vi "HapticSTM_raw.vi"() -> ()   [LabVIEW 2019]
uses:
  <userlib>/HapticSTM/HapticSTM.lvlib
  SubVIs/GlobalClicksHeight_raw.vi
  <userlib>/Nanonis Prog Interface V5/Nanonis Prog Interface.lvlib
panel:
  in  "Version?":bool
  in  "Setpoint (pA)":dbl=100.0
  in  "Depth (pA)":dbl=280.0
  in  "Shift (in)":dbl format="%.1f"
  in  "Hardness":dbl=0.7 format="%.1f"
  in  "Z Write?":bool
  out "function return":i32
  in  "Scaling?":bool
  out "Setpoint (pA)":dbl
  in  "Maximum (pA)":dbl=7000.0
  out "Filtered Current (pA)":dbl format="%.1f"
  out "Current (pA)":dbl format="%.1f"
  out "Oy":dbl
  out "Ox":dbl
  out "W":dbl
  out "H":dbl
  out "Z Write":dbl format="%^.1e"
  in  "Planing?":bool
  out "Button":bool
  out "Fy":dbl format="%.1f"
  out "Fz":dbl format="%.1f"
  out "Fx":dbl format="%.1f"
  out "x":dbl format="%.1f"
  out "y":dbl format="%.1f"
  out "z":dbl format="%0.1f"
  in  "Mode":u16(ring) items=["Log w/ Exp Z", "Log w/ Lin Z"]
  in  "Reset Clicks":bool
  out "Clicks":i32
  in  "STOP":bool
  in  "START":bool
  out "Seq":i32
  out "SeqString":string
  out "Raw and Scaled Z Positions":cluster{"X":dbl, "Y":dbl, "Z pen":dbl, "Z":dbl}(graph)
  out "Scaled Force and Current":T1(graph)
  # "Super Ultra Mega Haptic STM Controller 3000"
  # "Haptic Pen"
  # "Nanonis"
  # "Position"
  # "Z Controller"
  # "Force"
  # "Frame"
  # "Surface"
  # "Options"
  # "Addons"
  # "Test Data"
  # "Live"
  # "Small"
  # "Large"
  # "Current"
  # "No"
  # "Yes"
  # "Planing"
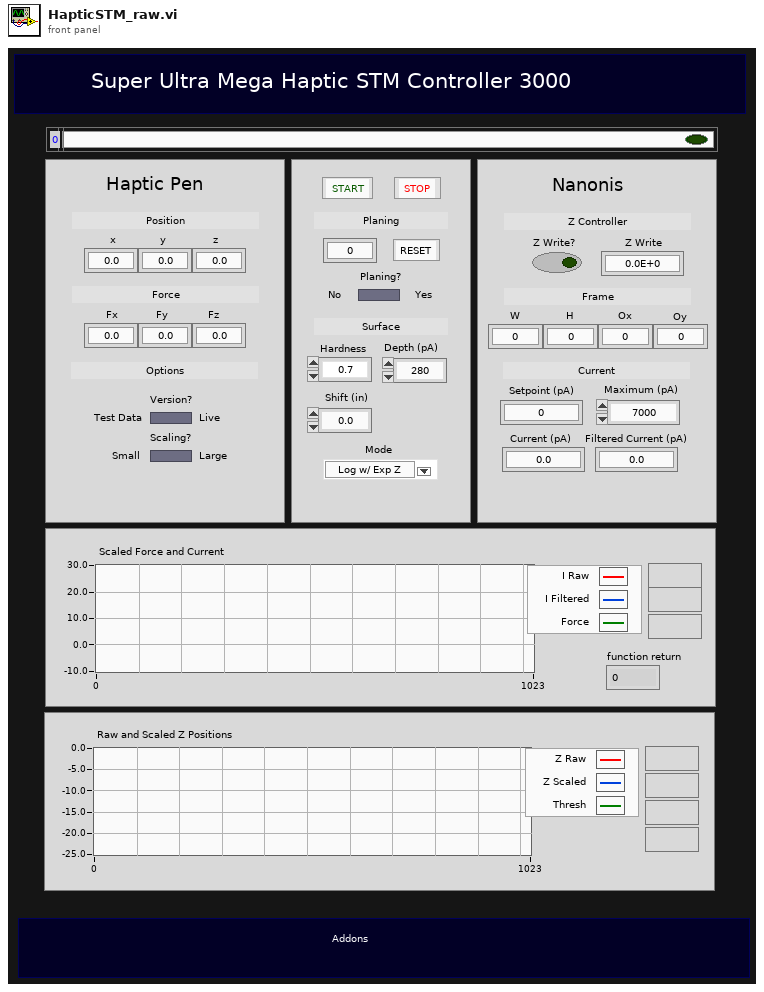
[diagram p1: front panel]
types:
  T1 = cluster{"Current (pA)":dbl, "Filtered Current (pA)":dbl, dbl}
  T2 = cluster{"Size (m)":cluster{"Width":sgl, "Height":sgl}, "Center coordinates (m)":cluster{"Xc":sgl, "Yc":sgl}}
  T3 = cluster{"Position":cluster{"X":dbl, "Y":dbl, "Zpen":dbl}, void, "y scaled (m)":dbl}
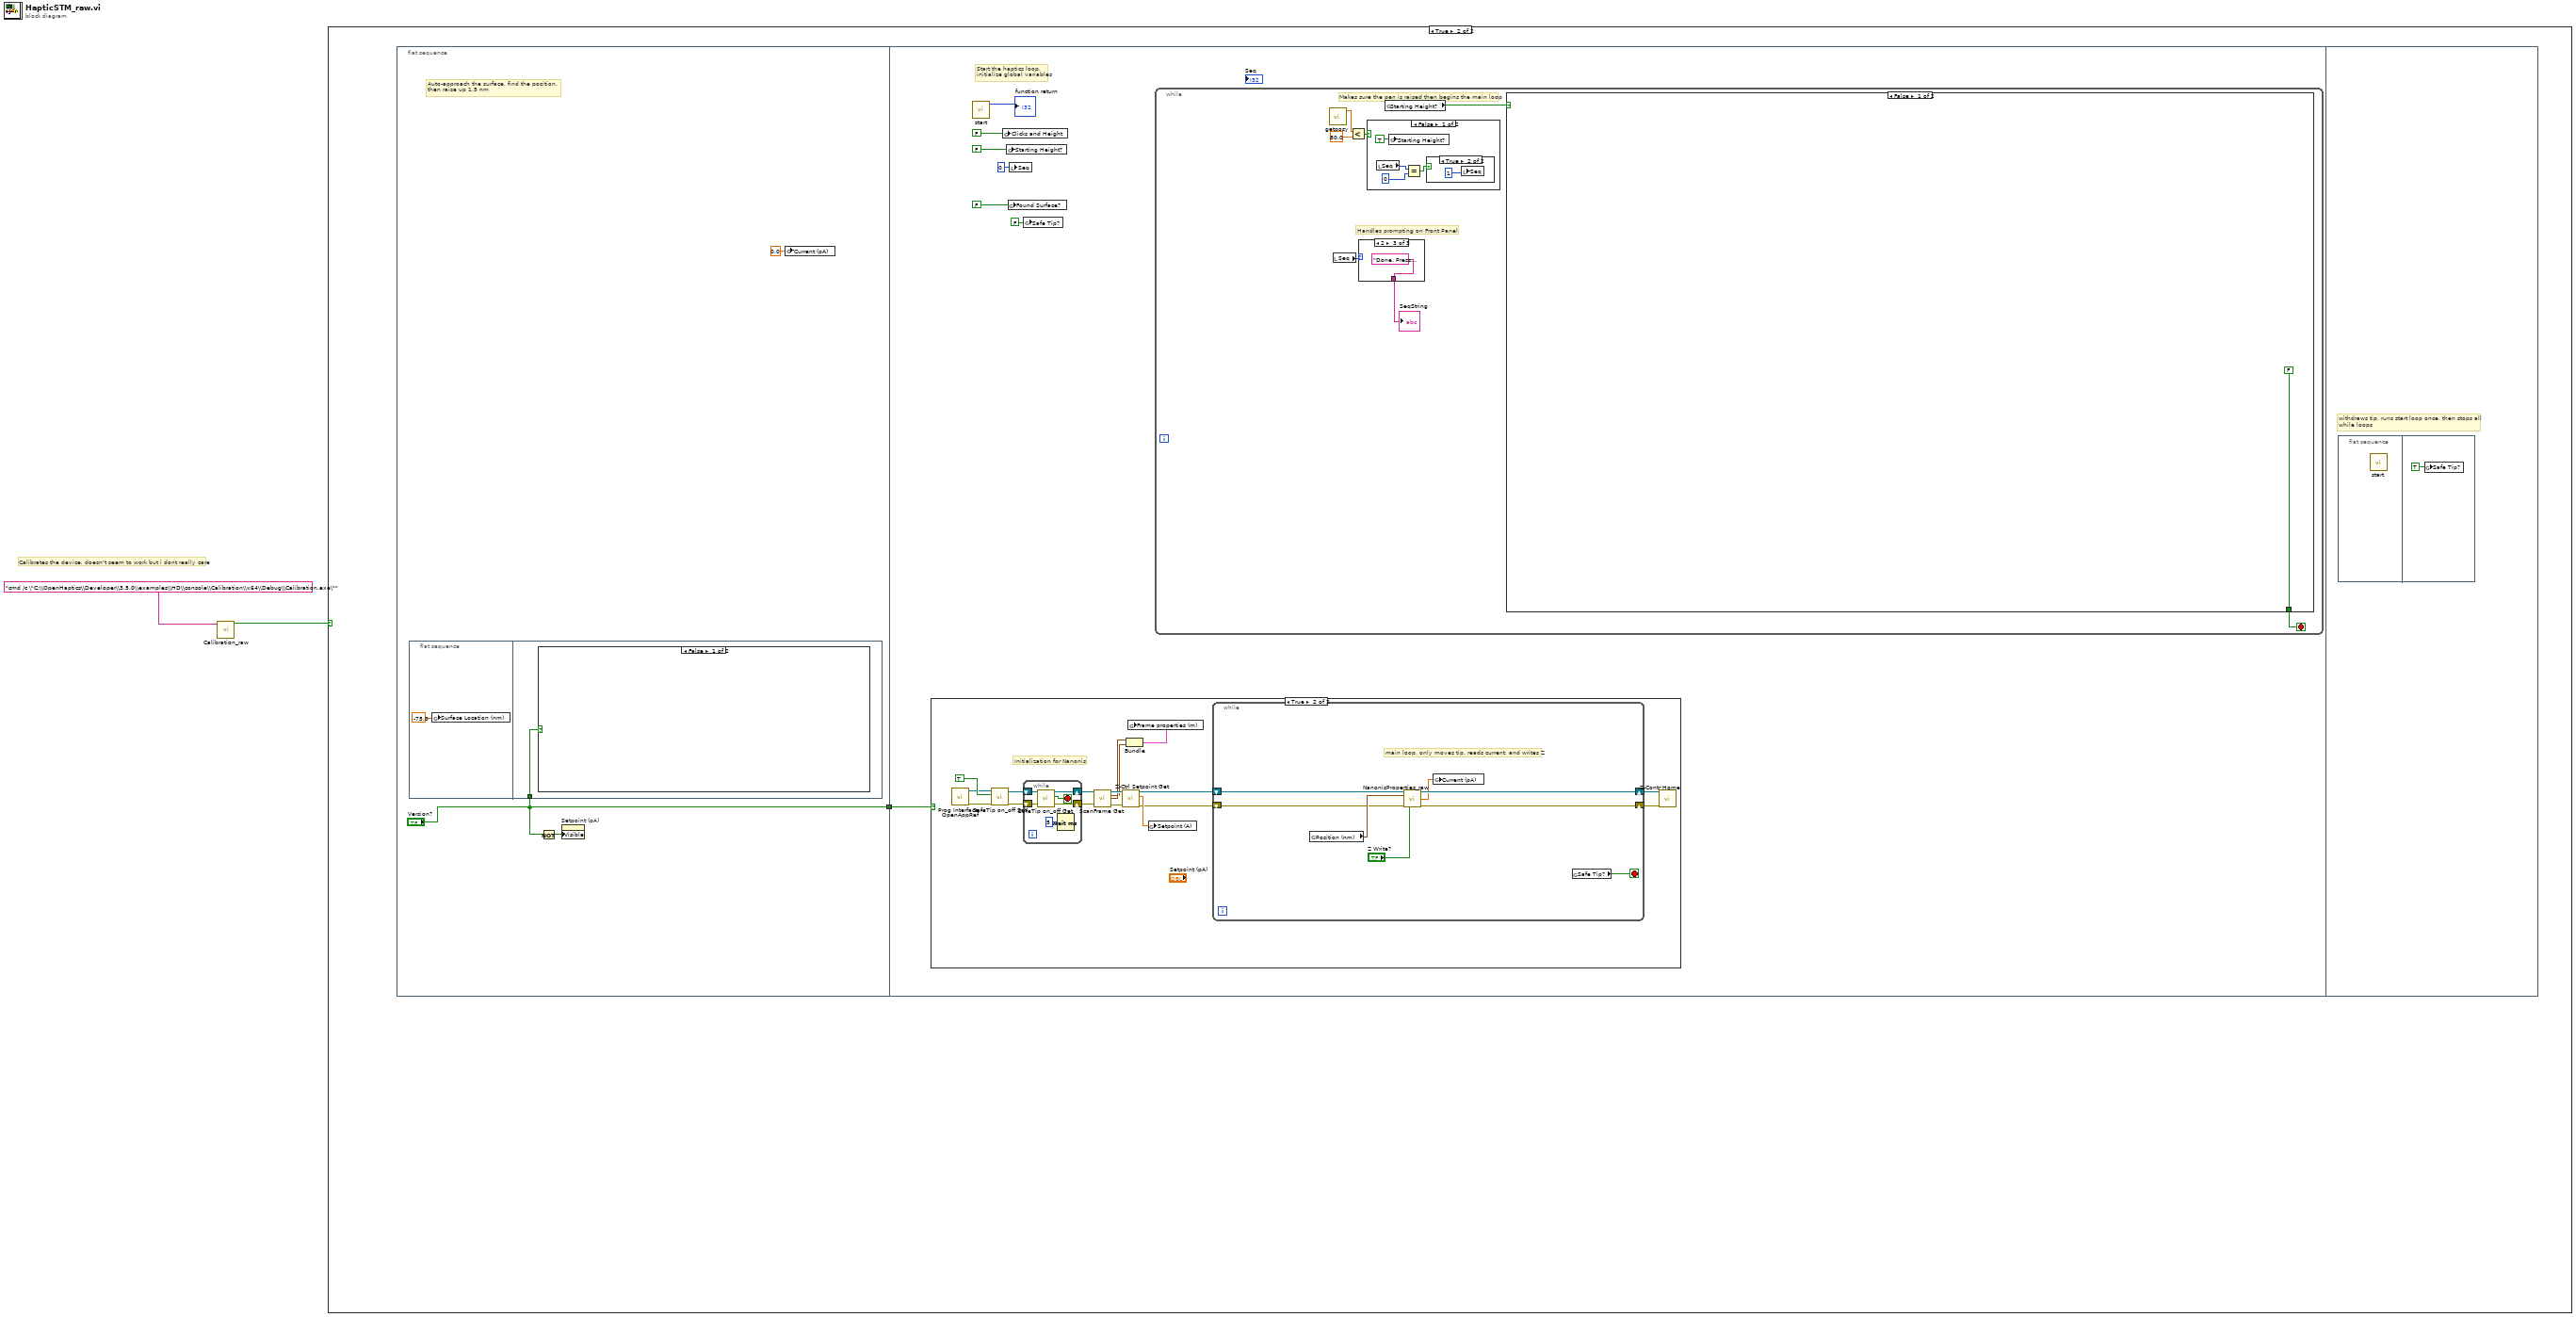
[diagram p0: block diagram]
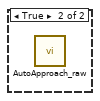
[diagram p3: hidden frame]
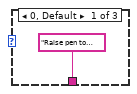
[diagram p5: hidden frame]
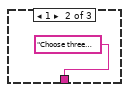
[diagram p6: hidden frame]
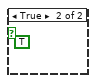
[diagram p8: hidden frame]
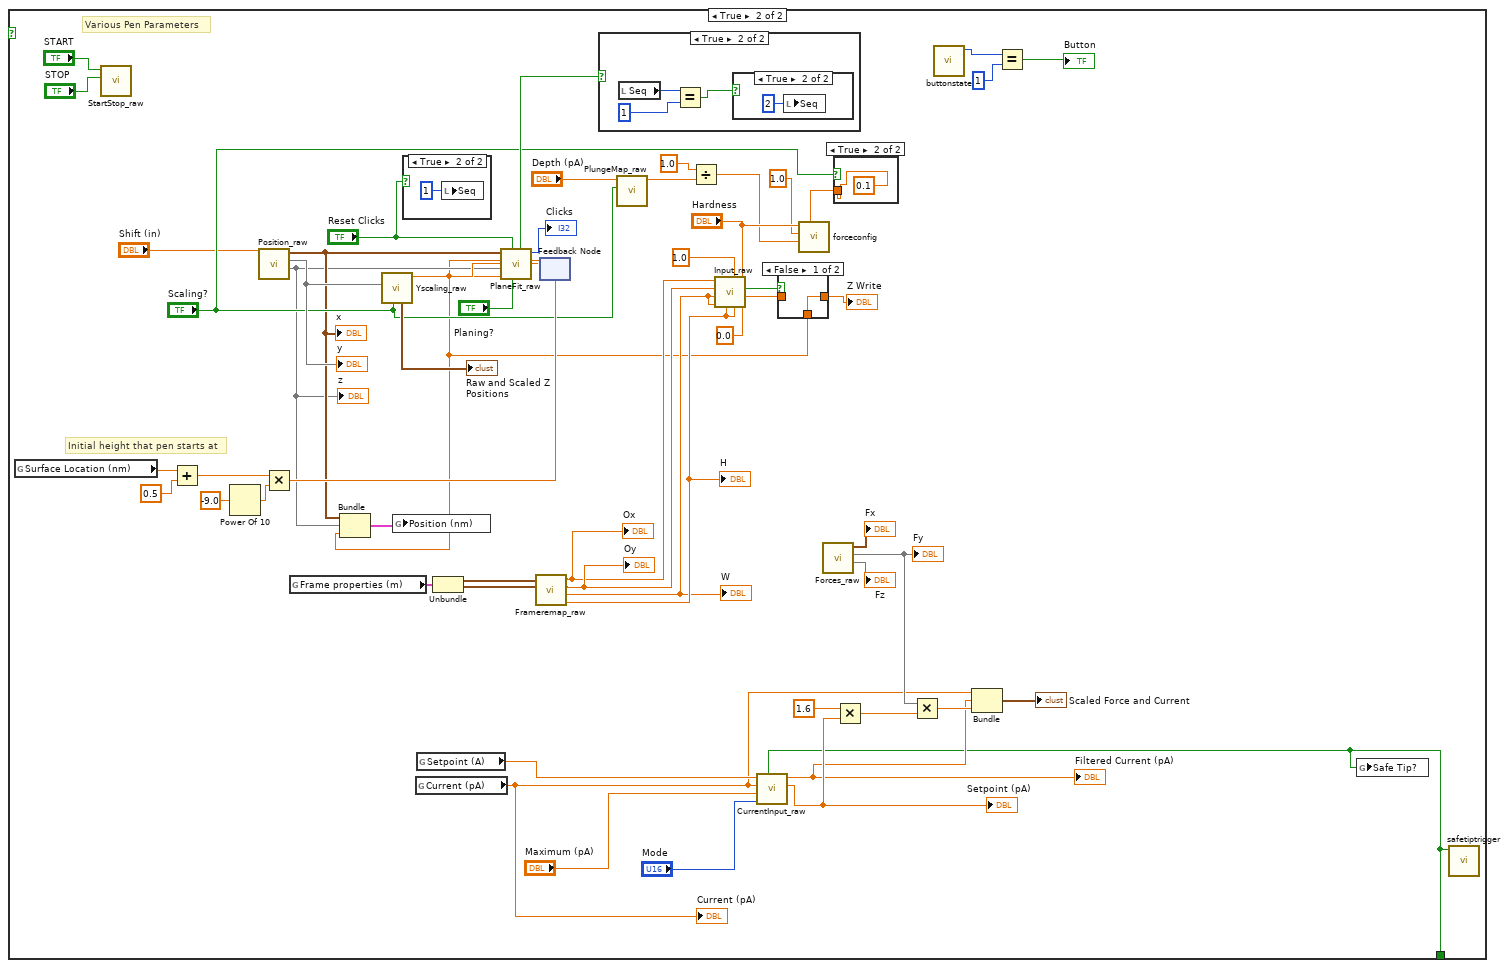
[diagram p9: hidden frame]
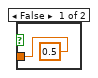
[diagram p10: hidden frame]
diagram:
  # "Calibrates the device, doesn't seem to work but i dont really care"
  n1 = call "Calibration_raw.vi"("command line"="cmd /c \"C:\\OpenHaptics\\Developer\\3.5.0\\examples\\HD\\console\\Calibration\\x64\\Debug\\Calibration.exe\"") -> ("Calibration Complete?"=w2:bool)  [unwired: 10 in]
  n2 = case shown="True" w2 {
    frame False {
    }
    frame True {
      n3 = flat-sequence {
        tunnel: ["Version?"] -> w3
        tunnel: w3 -> [w9]
        frame #0 {
          # "Auto-approach the surface, find the position, \nthen raise up 1.5 nm"
          n4 = flat-sequence {
            tunnel: "Version?" -> [w8]
            frame #0 {
              n5 = global write "GlobalClicksHeight_raw.vi" "Surface Location (nm)"(-75.0 ("Surface Location")) -> ()
            }
            frame #1 {
              n6 = case shown="False" w8 {
                frame False {
                }
                frame True {
                  n7 = call "AutoApproach_raw.vi"() -> ()  [unwired: 12 in]
                }
              }
            }
          }
          n8 = Not(x="Version?") -> (.not. x?=w5:bool)
          n9 = property on="Setpoint (pA)" class="DigNum (strict)"("Visible"=w5) -> ()  [unwired: 2 in, 2 out]
          n10 = global write "GlobalClicksHeight_raw.vi" "Current (pA)"(0.0 ("Current (pA)")) -> ()
        }
        frame #1 {
          # "Start the haptics loop,\ninitialize global variables"
          n11 = case shown="True" w9 {
            frame False {
            }
            frame True {
              # "Initialization for Nanonis"
              n12 = call <userlib>:"Prog Interface - OpenAppRef.vi"() -> ("Error out"=w30:errorcluster, "Application reference"=w31:refnum<vi>)  [unwired: 6 in]
              n13 = call <userlib>:"SafeTip on_off Set.vi"("error in (no error)"=w30, "SafeTip ON/OFF"=TRUE, "Application ref in"=w31) -> ("error out"=w28:errorcluster, "Application ref out"=w29:refnum<vi>)  [unwired: 7 in]
              n14 = while {
                shift-right: [w35] -> w27
                shift-left: w29 -> [w37]
                shift-right: [w34] -> w26
                shift-left: w28 -> [w36]
                stop <- w38 stop-if-true
                n15 = call <userlib>:"SafeTip on_off Get.vi"("error in (no error)"=w36, "Application ref in"=w37) -> ("error out"=w34:errorcluster, "SafeTip on/off status"=w38:bool, "Application ref out"=w35:refnum<vi>)  [unwired: 7 in]
                n16 = Wait (ms)(milliseconds to wait=u32 5) -> ()  [unwired: 1 out]
              }
              n17 = call <userlib>:"ScanFrame Get.vi"("Application ref in"=w27, "error in (no error)"=w26) -> ("Application ref out"=w25:refnum<vi>, "Center coordinates (m)"=w16:cluster{"Xc":sgl, "Yc":sgl}, "Size (m)"=w17:cluster{"Width":sgl, "Height":sgl}, "error out"=w24:errorcluster)  [unwired: 9 in, 1 out]
              n18 = call <userlib>:"Z-Ctrl Setpoint Get.vi"("error in (no error)"=w24, "Application ref in"=w25) -> ("error out"=w21:errorcluster, "Z Controller setpoint"=w23:sgl, "Application ref out"=w22:refnum<vi>)  [unwired: 6 in]
              n19 = Bundle("Size (m)"=w17, "Center coordinates (m)"=w16) -> (w18:T2)  [unwired: 1 in]
              n20 = global write "GlobalClicksHeight_raw.vi" "Frame properties (m)"(w18) -> ()
              n21 = global write "GlobalClicksHeight_raw.vi" "Setpoint (A)"(w23) -> ()
              n22 = while {
                shift-right: [w40] -> w19
                shift-left: w21 -> [w42]
                shift-right: [w41] -> w20
                shift-left: w22 -> [w44]
                stop <- w46 stop-if-true
                # "main loop, only moves tip, reads current, and writes Z"
                n23 = global read "GlobalClicksHeight_raw.vi" "Position (nm)"() -> (w45:cluster{"X":dbl, "Z":dbl, "Y":dbl})
                n24 = call "NanonisProperties_raw.vi"("Application ref in"=w44, "Position (nm)"=w45, "error in (no error)"=w42, "Z Write?"="Z Write?") -> ("Application ref out"=w41:refnum<vi>, "Current (pA)"=w39:sgl, "error out"=w40:errorcluster)  [unwired: 9 in]
                n25 = global write "GlobalClicksHeight_raw.vi" "Current (pA)"(w39) -> ()
                n26 = global read "GlobalClicksHeight_raw.vi" "Safe Tip?"() -> (w46:bool)
              }
              n27 = call <userlib>:"Z-Contr Home.vi"("Error in (no error)"=w19, "Application ref in"=w20) -> ()  [unwired: 8 in, 2 out]
            }
          }
          n28 = call <userlib>:"start.vi"() -> ("function return"=→"function return":i32)  [unwired: 11 in]
          n29 = global write "GlobalClicksHeight_raw.vi" "Clicks and Height"(FALSE ("Clicks and Height")) -> ()
          n30 = global write "GlobalClicksHeight_raw.vi" "Starting Height?"(FALSE ("Clicks and Height")) -> ()
          n31 = global write "GlobalClicksHeight_raw.vi" "Found Surface?"(FALSE ("Clicks and Height")) -> ()
          n32 = local write "Seq"(0 ("Seq")) -> ()
          n33 = global write "GlobalClicksHeight_raw.vi" "Safe Tip?"(FALSE ("Safe Tip?")) -> ()
          n34 = while {
            stop <- w47 stop-if-true
            # "Makes sure the pen is raised then begins the main loop"
            # "Handles prompting on Front Panel"
            n35 = call <userlib>:"getposy.vi"() -> ("function return"=w53:dbl)  [unwired: 11 in]
            n36 = local read "Seq"() -> (w49:i32)
            n37 = Less?(x=w53, y=80.0) -> (x < y?=w51:bool)
            n38 = case shown="2" w49 {
              tunnel: ["Raise pen to begin." "Choose three points, then raise the arm to plane." "Done. Press 'STOP' to stop at anytime."] -> w48
              frame 0, Default {
              }
              frame 1 {
              }
              frame 2 {
              }
            }
            "SeqString" <- w48
            n39 = case shown="False" w51 {
              frame False {
                n40 = local read "Seq"() -> (w59:i32)
                n41 = global write "GlobalClicksHeight_raw.vi" "Starting Height?"(TRUE ("Starting Height?")) -> ()
                n42 = Equal?(x=w59, y=0) -> (x = y?=w57:bool)
                n43 = case shown="True" w57 {
                  frame False {
                  }
                  frame True {
                    n44 = local write "Seq"(1 ("Seq")) -> ()
                  }
                }
              }
              frame True {
                (unwired) TRUE ("Clicks and Height")
              }
            }
            n45 = global read "GlobalClicksHeight_raw.vi" "Starting Height?"() -> (w50:bool)
            n46 = case shown="False" w50 {
              tunnel: [FALSE ("Current Maxed?") w67] -> w47
              frame False {
              }
              frame True {
                # "Initial height that pen starts at"
                # "Various Pen Parameters"
                n47 = global read "GlobalClicksHeight_raw.vi" "Surface Location (nm)"() -> (w82:dbl)
                n48 = call "StartStop_raw.vi"("STOP"="STOP", "START"="START") -> ()  [unwired: 10 in]
                n49 = Add(x=w82, y=0.5) -> (x+y=w79:dbl)
                n50 = Power Of 10(x=-9.0) -> (10^x=w78:dbl)
                n51 = call "Position_raw.vi"("Shift"="Shift (in)") -> (1:w70, 2:w108, "Position"=w71:cluster{"X":dbl, "Y":dbl, "Zpen":dbl})  [unwired: 8 in]
                "x" <- w71
                "y" <- w108
                "z" <- w70
                n52 = Multiply(x=w79, y=w78) -> (x*y=w80:dbl)
                n53 = global read "GlobalClicksHeight_raw.vi" "Frame properties (m)"() -> (w66:cluster{cluster{dbl, dbl}, cluster{dbl, dbl}})
                n54 = case shown="True" "Reset Clicks" {
                  frame False {
                  }
                  frame True {
                    n55 = local write "Seq"(1 ("Seq")) -> ()
                  }
                }
                n56 = global read "GlobalClicksHeight_raw.vi" "Current (pA)"() -> (w63:dbl)
                "Current (pA)" <- w63
                n57 = global read "GlobalClicksHeight_raw.vi" "Setpoint (A)"() -> (w68:dbl)
                n58 = Unbundle(w66) -> (w65:cluster{dbl, dbl}, w64:cluster{dbl, dbl})
                n59 = call "Frameremap_raw.vi"("Frame Origin (m)"=w64, "Frame Size (m)"=w65) -> ("FH (nm)"=w92:dbl, "FW (nm)"=w91:dbl, "Z Origin (nm)"=w90:dbl, "X Origin (nm)"=w89:dbl)  [unwired: 6 in]
                "H" <- w92
                "W" <- w91
                "Ox" <- w89
                "Oy" <- w90
                n60 = feedback #1(w80) -> (w114:dbl)
                n61 = call "Yscaling_raw.vi"(6:"Scaling?", "Plane Height (m)"=w108, 11:w114) -> ("y scaled (m)"=w69:dbl, "Position"=→"Raw and Scaled Z Positions":cluster{"X":dbl, "Y":dbl, "Z pen":dbl, "Z":dbl})  [unwired: 6 in, 1 out]
                n62 = Bundle("Position"=w71, w70, "y scaled (m)"=w69) -> (w72:T3)  [unwired: 1 in]
                n63 = global write "GlobalClicksHeight_raw.vi" "Position (nm)"(w72) -> ()
                n64 = call "PlaneFit_raw.vi"("Planing y/n?"="Planing?", "Reset Clicks"="Reset Clicks", "Y PEN"=w69, "Z"=w70, "Nano Z"=w69, 11:w71) -> ("Plane Height (m)"=w115:dbl, "Clicks"=→"Clicks":i32, "Planing Done?"=w101:bool)  [unwired: 3 in]
                n65 = feedback-in #1(w115) -> ()
                n66 = case shown="True" w101 {
                  frame False {
                  }
                  frame True {
                    n67 = local read "Seq"() -> (w128:i32)
                    n68 = Equal?(x=w128, y=1) -> (x = y?=w126:bool)
                    n69 = case shown="True" w126 {
                      frame False {
                      }
                      frame True {
                        n70 = local write "Seq"(2 ("Seq")) -> ()
                      }
                    }
                  }
                }
                n71 = call "PlungeMap_raw.vi"("Scaling?"="Scaling?", "Input (pA)"="Depth (pA)") -> ("output"=w83:dbl)  [unwired: 9 in]
                n72 = Divide(x=1.0, y=w83) -> (x/y=w93:dbl)
                n73 = call "Input_raw.vi"("Current * 10^input"=0.0, "Sensitivity"="Hardness", 4:w92, "Drag"=1.0, 6:w92, 8:w91, 9:w91, 10:w90, "Frame Properties (Remapped)"=w89) -> ("Scaled Current"=w95:dbl, "feedback"=w97:bool)  [unwired: 1 in]
                n74 = call "CurrentInput_raw.vi"("Mode"="Mode", "Maximum (pA)"="Maximum (pA)", "Current (pA)"=w63, "Setpoint (A)"=w68) -> ("Setpoint (pA)"=w85:dbl, "Filtered Current (pA)"=w76:dbl, "Safetip?"=w67:bool)  [unwired: 5 in]
                "Filtered Current (pA)" <- w76
                "Setpoint (pA)" <- w85
                n75 = case shown="False" w97 {
                  tunnel: [w123 w124] -> w96
                  tunnel: w95 -> [_ w124]
                  tunnel: w69 -> [w123 _]
                  frame False {
                  }
                  frame True {
                  }
                }
                "Z Write" <- w96
                n76 = call "Forces_raw.vi"() -> (1:→"Fz", 2:w112, "Forces"=→"Fx":cluster{"Fy":dbl, "Fz":dbl, "Fx":dbl})  [unwired: 9 in]
                "Fy" <- w112
                n77 = case shown="True" "Scaling?" {
                  tunnel: [0.5 0.1] -> w75
                  frame False {
                  }
                  frame True {
                  }
                }
                n78 = call <userlib>:"forceconfig.vi"("spc"=w75, "c"=w93, "b"=1.0, "a"="Hardness") -> ()  [unwired: 8 in]
                n79 = Multiply(x=1.6 ("y"), y=w85) -> (x*y=w109:dbl)
                n80 = Multiply(x=w112, y=w109) -> (x*y=w111:dbl)
                n81 = call <userlib>:"buttonstate.vi"() -> ("function return"=w107:i32)  [unwired: 11 in]
                n82 = Bundle("Current (pA)"=w63, "Filtered Current (pA)"=w76, w111) -> (→"Scaled Force and Current":T1)  [unwired: 1 in]
                n83 = Equal?(x=w107, y=1) -> (x = y?=→"Button":bool)
                n84 = global write "GlobalClicksHeight_raw.vi" "Safe Tip?"(w67) -> ()
                n85 = call <userlib>:"safetiptrigger.vi"("triggered"=w67) -> ()  [unwired: 11 in]
              }
            }
          }
        }
        frame #2 {
          # "withdraws tip, runs start loop once, then stops all\nwhile loops"
          n86 = flat-sequence {
            frame #0 {
              n87 = call <userlib>:"start.vi"() -> ()  [unwired: 11 in, 1 out]
            }
            frame #1 {
              n88 = global write "GlobalClicksHeight_raw.vi" "Safe Tip?"(TRUE ("Safe Tip?")) -> ()
            }
          }
        }
      }
    }
  }
